vi "setColors.vi"(8 "error in (no error)":errorcluster, 10 "colors":string[](array[string]), 11 "Flightweight Pattern Demo in":refnum<class "Flightweight Pattern Demo.lvclass">) -> (0 "error out":errorcluster, 3 "Flightweight Pattern Demo out":refnum<class "Flightweight Pattern Demo.lvclass">)   [LabVIEW 2017, in "Flightweight Pattern Demo.lvclass"]
uses:
  Flightweight Pattern Demo.lvclass
  Flightweight Pattern Demo.lvclass/Flightweight Pattern Demo.ctl
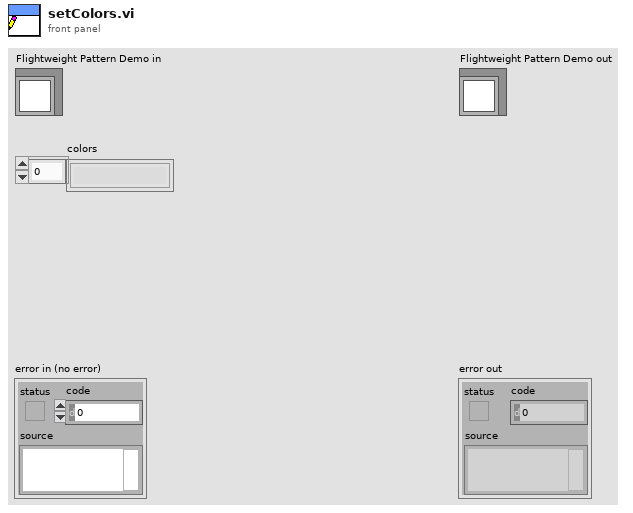
[diagram p1: front panel]
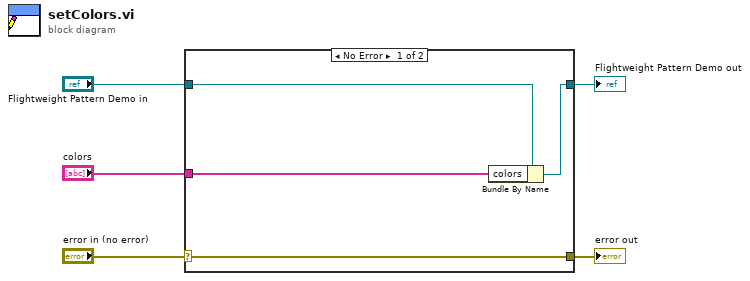
[diagram p0: block diagram]
diagram:
  n1 = case shown="No Error" "error in (no error)" {
    selector: "error in (no error)" -> [w9 w10]
    tunnel: [w9 w10] -> w4
    tunnel: [w7 w11] -> w2
    tunnel: "Flightweight Pattern Demo in" -> [w8 w11]
    tunnel: "colors" -> [w6 _]
    frame No Error {
      n2 = Bundle By Name(cluster=w8, "colors"=w6) -> (w7:refnum<class "Flightweight Pattern Demo.lvclass">)
    }
    frame Error {
    }
  }
  "error out" <- w4
  "Flightweight Pattern Demo out" <- w2
